vi "ODMR with B sweep.vi"() -> ()   [LabVIEW 2012]
uses:
  <vilib>/Utility/file.llb/Write To Spreadsheet File (DBL).vi
  <vilib>/Analysis/1siggen.llb/Ramp Pattern by Samples.vi
  <vilib>/Analysis/NI_AALBase.lvlib
panel:
  in  "p (dbm)":dbl=-4.0
  in  "Cluster":T1={"Freq start"=0.0, "Freq End"=0.0, "Freq Step"=0.0, "Power (dbm)"=0.0, "number of samples per channel"=-1}
  in  "low?":bool
  out "XY Graph":cluster{"Y":dbl[], "Y":dbl[]}[](graph)
  in  "samples":i32=25
  in  "End Mag V":dbl=2.5 format="%0.2f"
  in  "Start Mag V":dbl format="%0.2f"
  in  "file path (dialog if empty)":path=path "C:/Users/Ouyang Group/Documents/Data/7-12-16/MNP #2 wash CPW 5mW scan 2 x4 y131 T-63.2 d_1.55 "
  in  "Freq Sweep Cluster":T2={"GPIB address 2"="19", "resolution (10 Hz:2) 2"=2, "band (1-26.5:2) 2"=2, "Freq max"=4000000000.0, "Start Freq"=1000000000.0, "Freq Step"=0.02, "rate"=100.0, "samples per channel"=200} {"rate" format="%0.2f"; "resolution (10 Hz:2) 2" items=["0.1 Hz", "1 Hz", "10 Hz", "100 Hz", "1 KHz", "10 KHz", "100 KHz", "1 MHz", "10 MHz", "100 MHz", "1 GHz"]}
  in  "Dot Tracking Cluster":T3={"RS232 settings"={"Portnumber"=6, "Baudrate"=5}, "X Parameters"={"Number of X Steps"=200, "Max X (V)"=2.0, -2.0}, "Y Parameters"={"Number of Y Steps"=200, "Max Y (V)"=2.0, "Min Y (V)"=-2.0}, "X 89"=25.0, "Y Pos"=112.0, "Z Pos"=60.6, "Tracking interval"=150.0} {"RS232 settings"."Portnumber" items=["COM1", "COM2", "COM3", "COM4", "COM5", "COM6", "COM7", "COM8", "COM9", "COM10", "COM11", "COM12", "COM13", "COM14", "COM15", "COM16", "COM17", "COM18", "COM19", "COM20", "COM21", "COM22", "COM23", "COM24", "COM25", "COM26", "COM27", "COM28", "COM29", "COM30"]; "RS232 settings"."Baudrate" items=["9600", "14400", "19200", "38400", "57600", "115200"]}
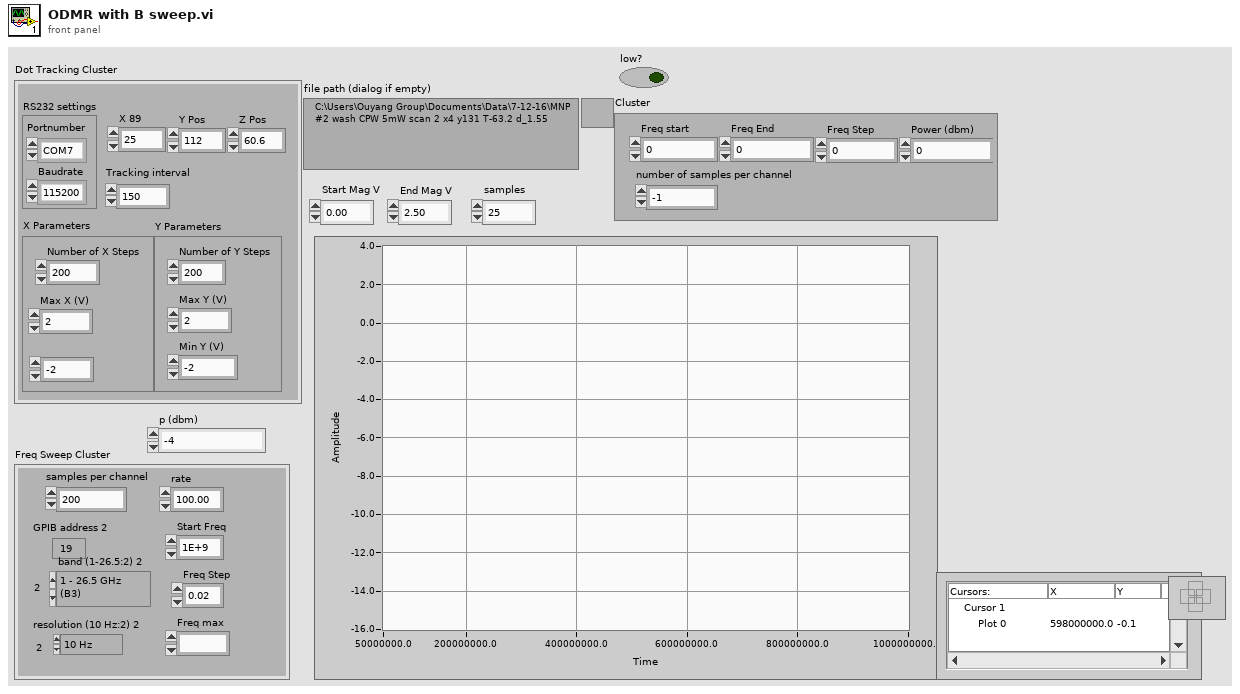
[diagram p1: front panel]
types:
  T1 = cluster{"Freq start":dbl, "Freq End":dbl, "Freq Step":dbl, "Power (dbm)":dbl, "number of samples per channel":i32}
  T2 = cluster{"GPIB address 2":string, "resolution (10 Hz:2) 2":i32, "band (1-26.5:2) 2":i32, "Freq max":ext, "Start Freq":dbl, "Freq Step":dbl, "rate":dbl, "samples per channel":i32}
  T3 = cluster{"RS232 settings":cluster{"Portnumber":i32, "Baudrate":u16}, "X Parameters":cluster{"Number of X Steps":i32, "Max X (V)":dbl, dbl}, "Y Parameters":cluster{"Number of Y Steps":i32, "Max Y (V)":dbl, "Min Y (V)":dbl}, "X 89":dbl, "Y Pos":dbl, "Z Pos":dbl, "Tracking interval":dbl}
  T4 = cluster{"Number of X Steps":i32, "Max X (V)":dbl, dbl}
  T5 = cluster{"Number of Y Steps":i32, "Max Y (V)":dbl, "Min Y (V)":dbl}
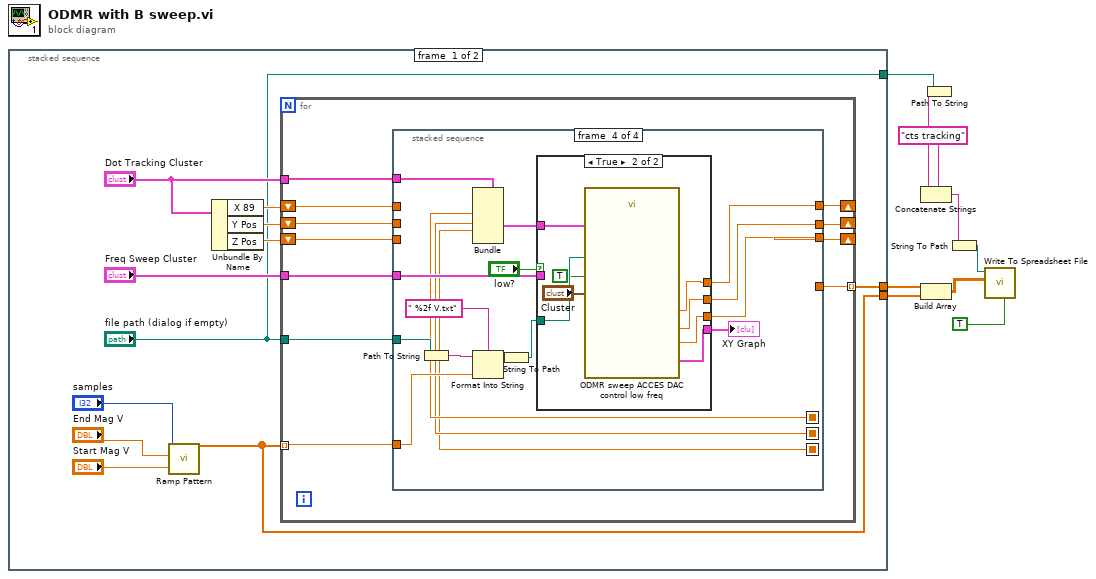
[diagram p0: block diagram]
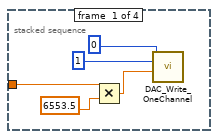
[diagram p2: hidden frame]
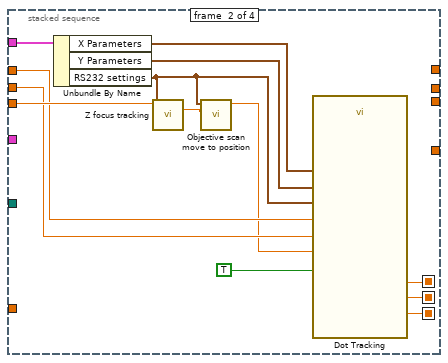
[diagram p3: hidden frame]
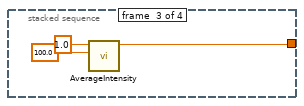
[diagram p4: hidden frame]
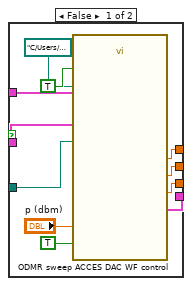
[diagram p5: hidden frame]
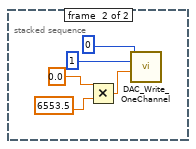
[diagram p6: hidden frame]
diagram:
  n1 = stacked-sequence {
    tunnel: [w12 _] -> w9
    tunnel: [w11 _] -> w8
    tunnel: ["file path (dialog if empty)" _] -> w5
    frame #0 {
      n2 = call-poly <vilib>:"Ramp Pattern.vi"("start"="Start Mag V", "end"="End Mag V", "samples"="samples") -> ("Ramp Pattern"=w11:dbl[])  [unwired: 7 in, 1 out]
      n3 = Unbundle By Name("Dot Tracking Cluster") -> ("X 89"=w16:dbl, "Y Pos"=w15:dbl, "Z Pos"=w14:dbl)
      n4 = for {
        tunnel: w11 -> [w22] mode=indexing
        tunnel: "Dot Tracking Cluster" -> [w31]
        shift-right: [w27] -> _
        shift-left: w16 -> [w30]
        shift-right: [w26] -> _
        shift-left: w15 -> [w29]
        shift-right: [w25] -> _
        shift-left: w14 -> [w28]
        tunnel: "Freq Sweep Cluster" -> [w24]
        tunnel: "file path (dialog if empty)" -> [w23]
        tunnel: [w21] -> w12 mode=indexing
        n5 = stacked-sequence {
          seq-local: [_ w41 _ _] -> [_ _ _ w59]
          seq-local: [_ w43 _ _] -> [_ _ _ w58]
          seq-local: [_ w42 _ _] -> [_ _ _ w57]
          tunnel: w31 -> [_ w49 _ w69]
          tunnel: w30 -> [_ w46 _ _]
          tunnel: w29 -> [_ w45 _ _]
          tunnel: w28 -> [_ w48 _ _]
          tunnel: [_ _ _ w67] -> w27
          tunnel: [_ _ _ w66] -> w26
          tunnel: [_ _ _ w65] -> w25
          tunnel: w24 -> [_ _ _ w64]
          tunnel: w23 -> [_ _ _ w63]
          tunnel: w22 -> [w36 _ _ w62]
          tunnel: [_ _ w50 _] -> w21
          frame #0 {
            n6 = Multiply(x=w36, y=6553.5) -> (x*y=w34:dbl)
            n7 = call "DAC_Write_OneChannel.vi"("Value"=w34, "Channel"=u16 1, "DeviceIndex"=u64 0) -> ()  [unwired: 7 in, 2 out]
          }
          frame #1 {
            n8 = Unbundle By Name(w49) -> ("X Parameters"=w47:T4, "Y Parameters"=w40:T5, "RS232 settings"=w39:cluster{"Portnumber":i32, "Baudrate":u16})
            n9 = call "Z focus tracking.vi"("Position"=w48, "RS232 settings"=w39) -> ("center"=w38:dbl)  [unwired: 6 in, 2 out]
            n10 = call "Objective scan move to position.vi"("Z position"=w38, "RS232 settings"=w39) -> ("Z Position 2"=w37:dbl)  [unwired: 9 in]
            n11 = call "Dot Tracking.vi"("X"=w47, "Y Parameters"=w40, "RS232 settings"=w39, "X Pos"=w46, "Y pos"=w45, "Z Pos"=w37, "Z-track?"=TRUE) -> ("X Position"=w41:dbl, "Y Position"=w43:dbl, "Z Position"=w42:dbl)  [unwired: 2 in, 4 out]
          }
          frame #2 {
            n12 = call "AverageIntensity.vi"("rate (Hz)"=100.0, "Time Target (s)"=1.0) -> ("Average intensity (cts/s)"=w50:dbl)  [unwired: 8 in, 1 out]
          }
          frame #3 {
            n13 = Path To String(path=w63) -> (string=w61:string)
            n14 = Bundle(cluster=w69, "X 89"=w59, "Y Pos"=w58, "Z Pos"=w57) -> (w68:T3)  [unwired: 4 in]
            n15 = Format Into String(format string=" %2f V.txt", initial string=w61, w62) -> (resulting string=w54:string)  [unwired: 1 in, 1 out]
            n16 = String To Path(string=w54) -> (path=w53:path)
            n17 = case shown="True" "low?" {
              tunnel: w68 -> [w80 w88]
              tunnel: [w79 w84] -> w67
              tunnel: [w78 w83] -> w66
              tunnel: [w77 w82] -> w65
              tunnel: w64 -> [w76 _]
              tunnel: [w75 w81] -> w56
              tunnel: w53 -> [w73 w87]
              frame False {
                n18 = call "ODMR sweep ACCES DAC WF control.vi"("leveling file"=path "C:/Users/Ouyang Group/Documents/Data/8-26-16/Windfreak plus switches and amp power calibration high res", "p (dbm)"="p (dbm)", "leveling"=TRUE, "Save?"=TRUE, "file path (dialog if empty)"=w73, "Freq Sweep Cluster"=w76, "Dot Tracking Cluster"=w80) -> ("Z Position"=w77:dbl, "Y Position"=w78:dbl, "X Position"=w79:dbl, "XY Graph"=w75:cluster{"Y":dbl[], "Y":dbl[]}[])  [unwired: 1 out]
              }
              frame True {
                n19 = call "ODMR sweep ACCES DAC control low freq.vi"("Save?"=TRUE, "file path (dialog if empty)"=w87, "Cluster"="Cluster", "Dot Tracking Cluster"=w88) -> ("Z Position"=w82:dbl, "Y Position"=w83:dbl, "X Position"=w84:dbl, "XY Graph"=w81:cluster{"Y":dbl[], "Y":dbl[]}[])  [unwired: 3 in, 1 out]
              }
            }
            "XY Graph" <- w56
          }
        }
      }
    }
    frame #1 {
      n20 = Multiply(x=0.0, y=6553.5) -> (x*y=w91:dbl)
      n21 = call "DAC_Write_OneChannel.vi"("Value"=w91, "Channel"=u16 1, "DeviceIndex"=u64 0) -> ()  [unwired: 7 in, 2 out]
    }
  }
  n22 = Build Array(w9, w8) -> (w7:dbl[][])
  n23 = Path To String(path=w5) -> (string=w4:string)
  n24 = Concatenate Strings(w4, "cts tracking" ("string")) -> (w2:string)
  n25 = String To Path(string=w2) -> (path=w1:path)
  n26 = call-poly <vilib>:"Write To Spreadsheet File.vi"("transpose? (no:F)"=TRUE, "2D data"=w7, "file path (dialog if empty)"=w1) -> ()  [unwired: 5 in, 1 out]
